vi "Begin stream Send.vi"(6 "contextId":T2, 8 "error in":errorcluster, 9 "timeout (ms)":i32=-1, 10 "Request Data":T3, 11 "gRPC ID":T2) -> (0 "error out":errorcluster, 2 "Optimized Streaming":T1, 3 "gRPC ID out":T2)   [LabVIEW 2021, in "streamtest_client.lvlib"]
uses:
  streamtest_client.lvlib
  <vilib>/gRPC/LabVIEW gRPC Library/Shared/grpcId.ctl
  RPC Messages/streamtest_Empty.ctl
  Optimized Streaming/typedef/Call ID.ctl
  59bd46bd-855a-43b3-a0b3-6a244c6a481b.vi
  <vilib>/gRPC/LabVIEW gRPC Library/Shared/TranslateGrpcError.vi
  <vilib>/gRPC/LabVIEW gRPC Library/Server API/Server/Get Server DLL Path.vi
  <vilib>/Utility/error.llb/Error Cluster From Error Code.vi
  <vilib>/gRPC/LabVIEW gRPC Library/grpc-lvsupport-release.lvlib
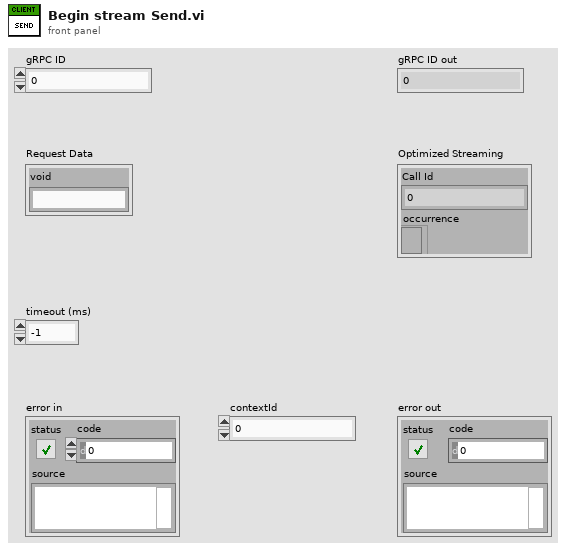
[diagram p1: front panel]
types:
  T1 = typedef "Call ID.ctl" = cluster{"Call Id":T2, "occurrence":refnum<k4>}
  T2 = typedef "grpc-lvsupport-release.lvlib/grpcId.ctl" = u64
  T3 = typedef "streamtest_client.lvlib/streamtest_Empty.ctl" = cluster{"void":string}
  T4 = typedef "streamtest_client.lvlib/streamtest_Empty_Flat.ctl" = cluster{"void":string}
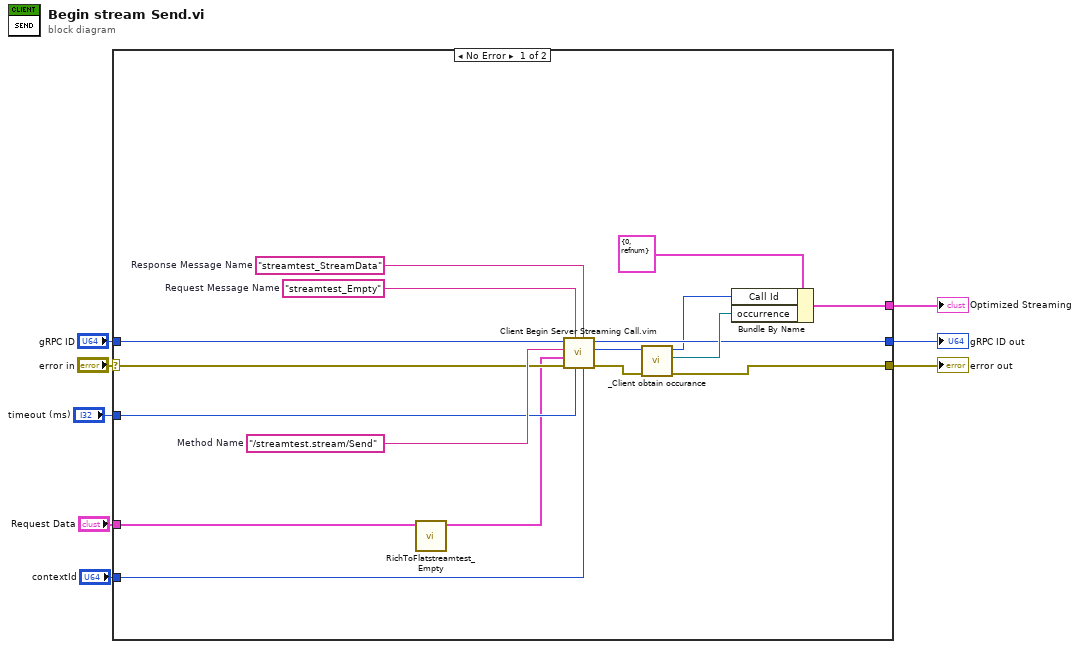
[diagram p0: block diagram]
diagram:
  n1 = case shown="No Error" "error in" {
    selector: "error in" -> [w22 w26]
    tunnel: [w15 w26] -> w7
    tunnel: "gRPC ID" -> [w21 w27]
    tunnel: [w11 w27] -> w5
    tunnel: "Request Data" -> [w18 _]
    tunnel: "timeout (ms)" -> [w20 _]
    tunnel: "contextId" -> [w19 _]
    tunnel: [w12 _] -> w1
    frame No Error {
      w23 = "streamtest_StreamData"  # Response Message Name
      w24 = "streamtest_Empty"  # Request Message Name
      w25 = "/streamtest.stream/Send"  # Method Name
      n2 = call "RichToFlatstreamtest_Empty.vi"("InputCluster"=w18) -> ("OutputCluster"=w17:T4)  [unwired: 10 in]
      n3 = call "Client Begin Server Streaming Call.vim"("contextId"=w19, "Response Message Name"=w23, "timeout (ms)"=w20, "Request Message Name"=w24, "error in"=w22, "Request Data"=w17, "Method Name"=w25, "ClientID in"=w21) -> ("error out"=w16:errorcluster, "Call ID out"=w10:u64, "ClientID out"=w11:u64)  [unwired: 1 in]
      n4 = call "_Client obtain occurance.vi"("error in"=w16, "Call ID in"=w10) -> ("error out"=w15:errorcluster, "occurrence"=w13:refnum<k4>, "Call ID out"=w9:T2)  [unwired: 7 in]
      n5 = Bundle By Name(cluster=T1 {"Call Id"=0, "occurrence"=refnum} ("Optimized Streaming"), "Call Id"=w9, "occurrence"=w13) -> (w12:T1)
    }
    frame Error {
    }
  }
  "error out" <- w7
  "gRPC ID out" <- w5
  "Optimized Streaming" <- w1
